vi "4Pi PR.vi"(7 "Calling VI Ref":refnum<vi>) -> ()   [LabVIEW 2021]
uses:
  <vilib>/Utility/miscctls.llb/LVPointTypeDef.ctl
  4Pi Dual DM Control/4Pi Dual DM - Controls/4Pi Dual DM - Standard Action.ctl
  <vilib>/Utility/file.llb/Read Delimited Spreadsheet (DBL).vi
panel:
  in  "Update DM":bool
  out "Spherical":sgl=1.0 format="%.3g"
  out "Coma (x)":sgl=1.0 format="%.3g"
  out "Coma (y)":sgl=1.0 format="%.3g"
  out "Astigmatsim":sgl=1.0 format="%.3g"
  out "Astigmatsim (diag)":sgl=1.0 format="%.3g"
  out "phase plot":cluster{u16[], sgl[]}(graph)
  in  "p factor":dbl=1.0
  in  "Quit":bool
  in  "Start PR":bool
  in  "objective":u16(ring) items=["Bottom", "Top"]
  in  "channel":u16(ring) items=["600", "676"]
  in  "gain":dbl=2.0
  in  "CCD offset":dbl=100.0
  in  "z range (µm)":dbl[](array[numeric])=[-1.0, 1.0, 0.2]
  in  "pixel size  (µm)":dbl=0.129
  in  "refractive index":dbl=1.406
  in  "NA":dbl=1.35
  # "z (µm)[start, end, step]"
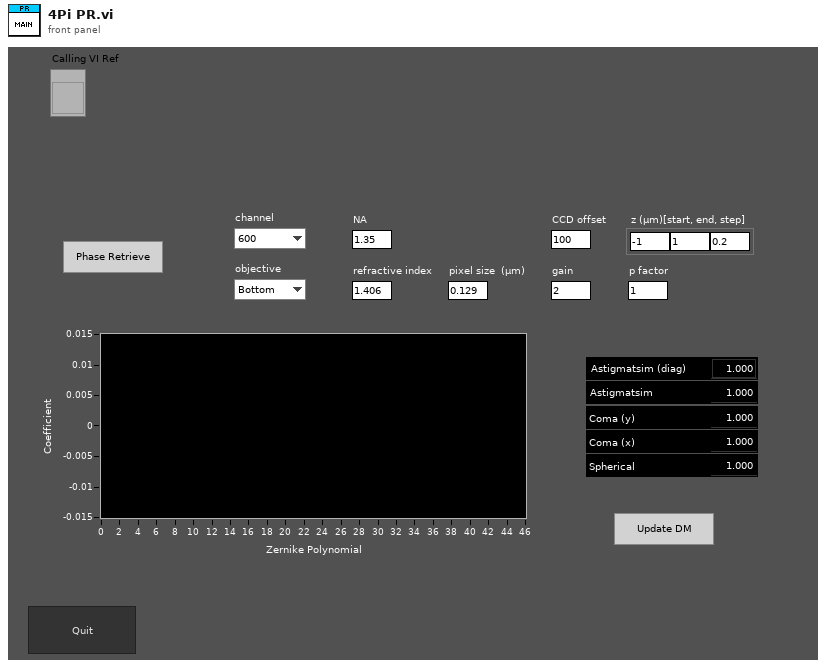
[diagram p1: front panel]
types:
  T1 = enum16{"Always On", "Always Off", "Off While Running"}
  T2 = typedef "LVPointTypeDef.ctl" = cluster{"Horizontal":i16, "Vertical":i16}
  T3 = typedef "4Pi Dual DM - Standard Action.ctl" = enum16{"Read", "Write"}
  T4 = typedef "4Pi Dual DM - Mirror Modes DUAL.ctl" = cluster{"Mode":string, "Amplitude":dbl}[][]
  T5 = typedef "LVRectTypeDef.ctl" = cluster{"Left":i16, "Top":i16, "Right":i16, "Bottom":i16}
  T6 = typedef "LVBoundsTypeDef.ctl" = cluster{"Width":u32, "Height":u32}
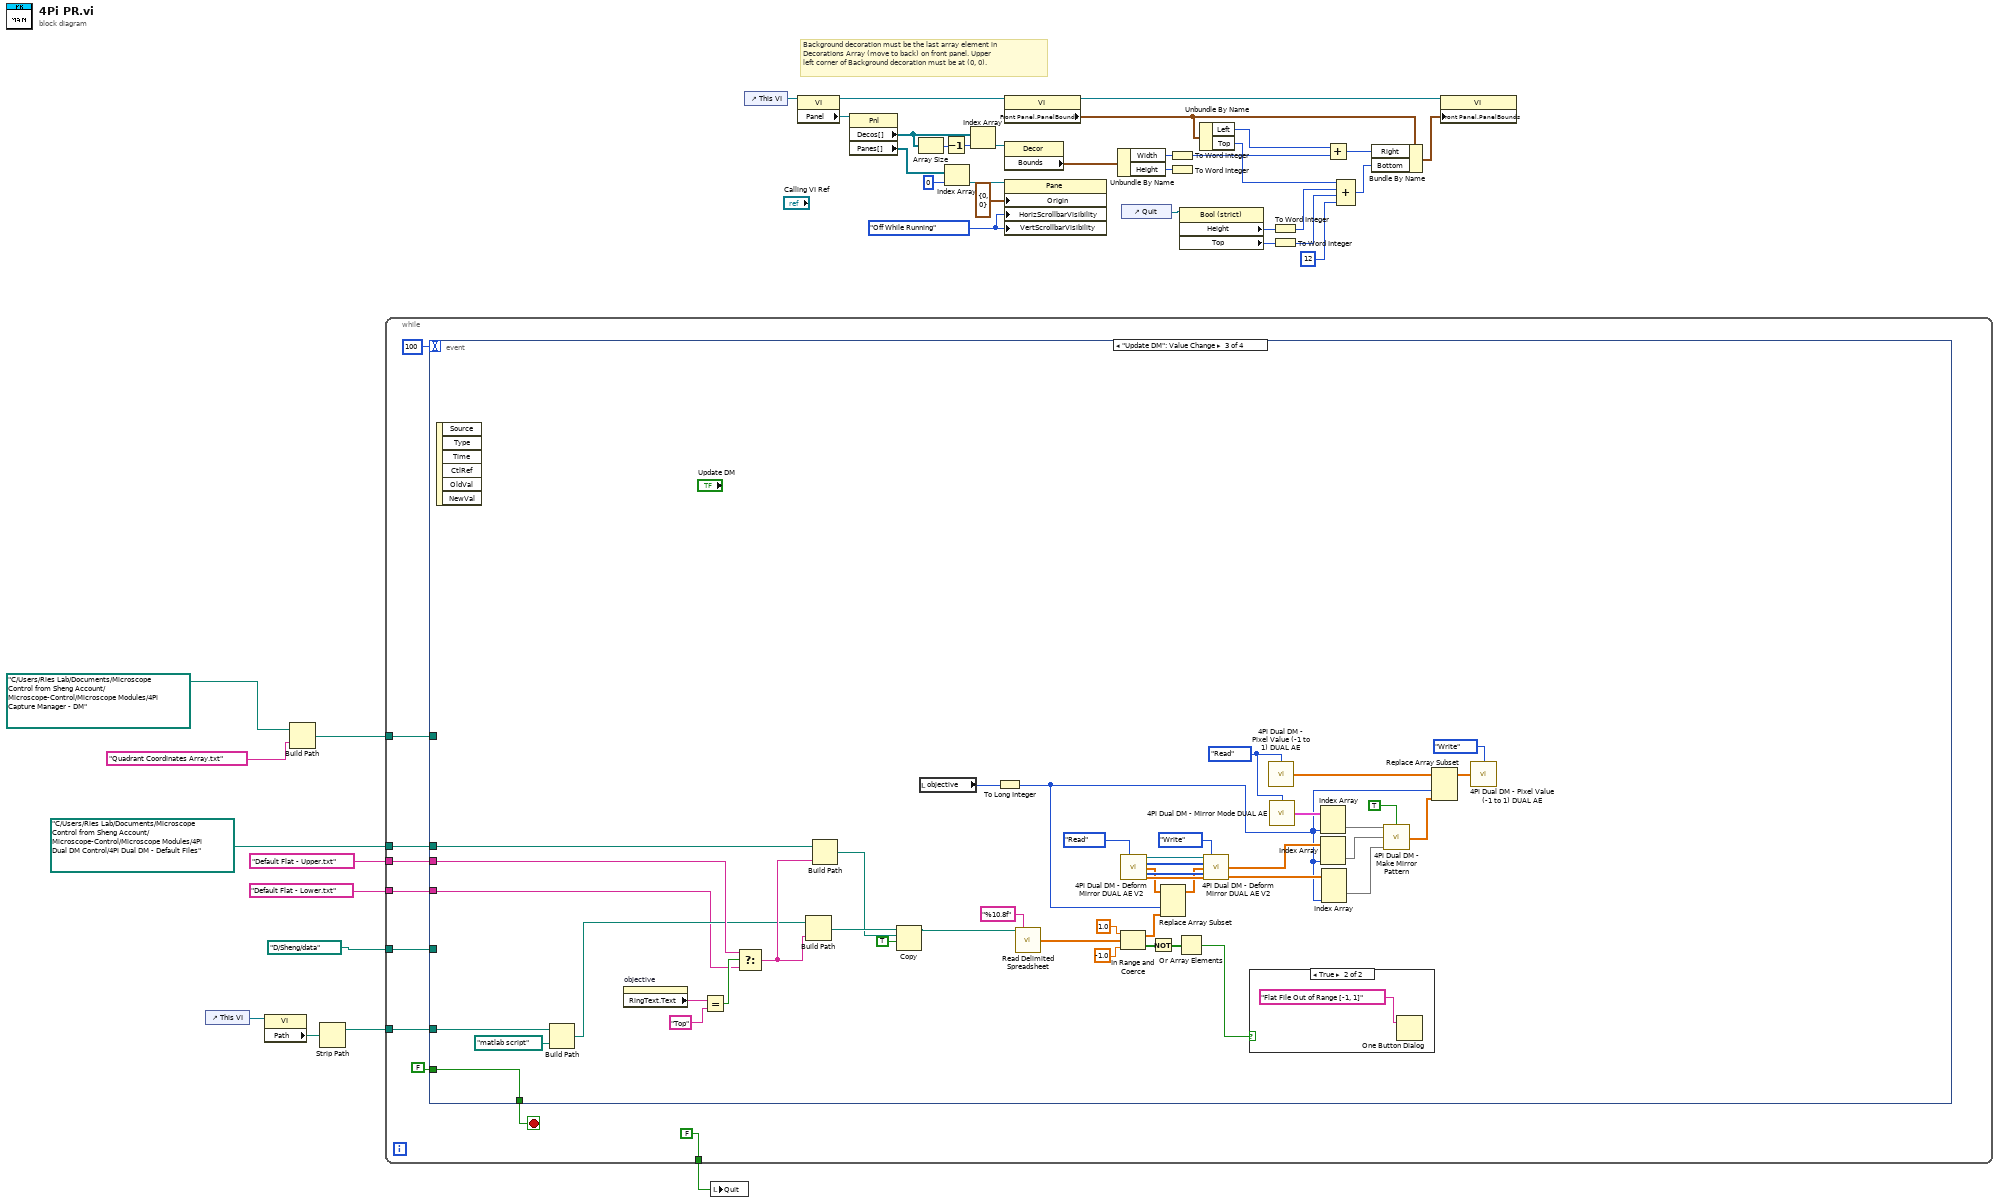
[diagram p0: block diagram]
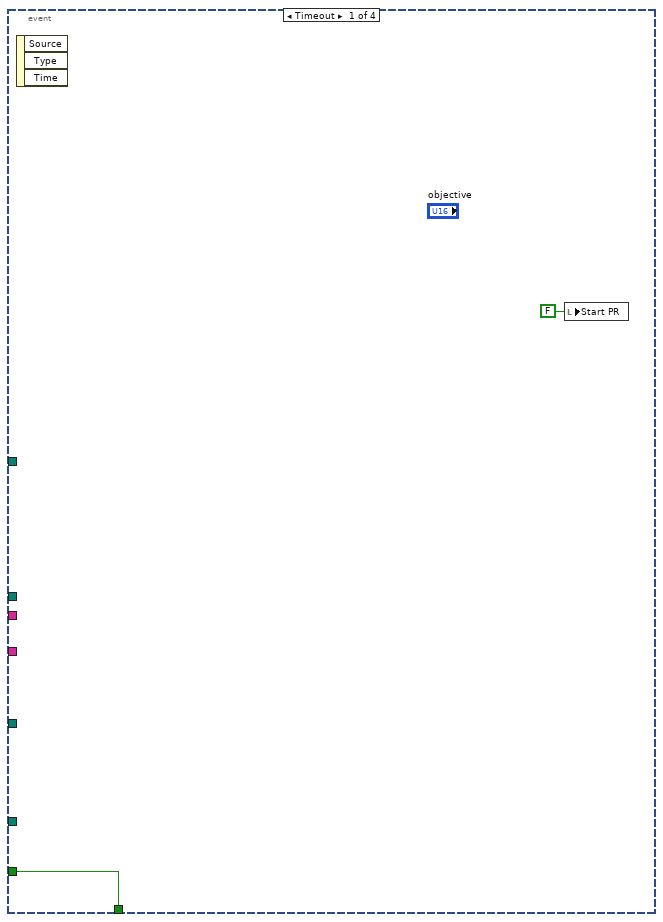
[diagram p2: hidden frame]
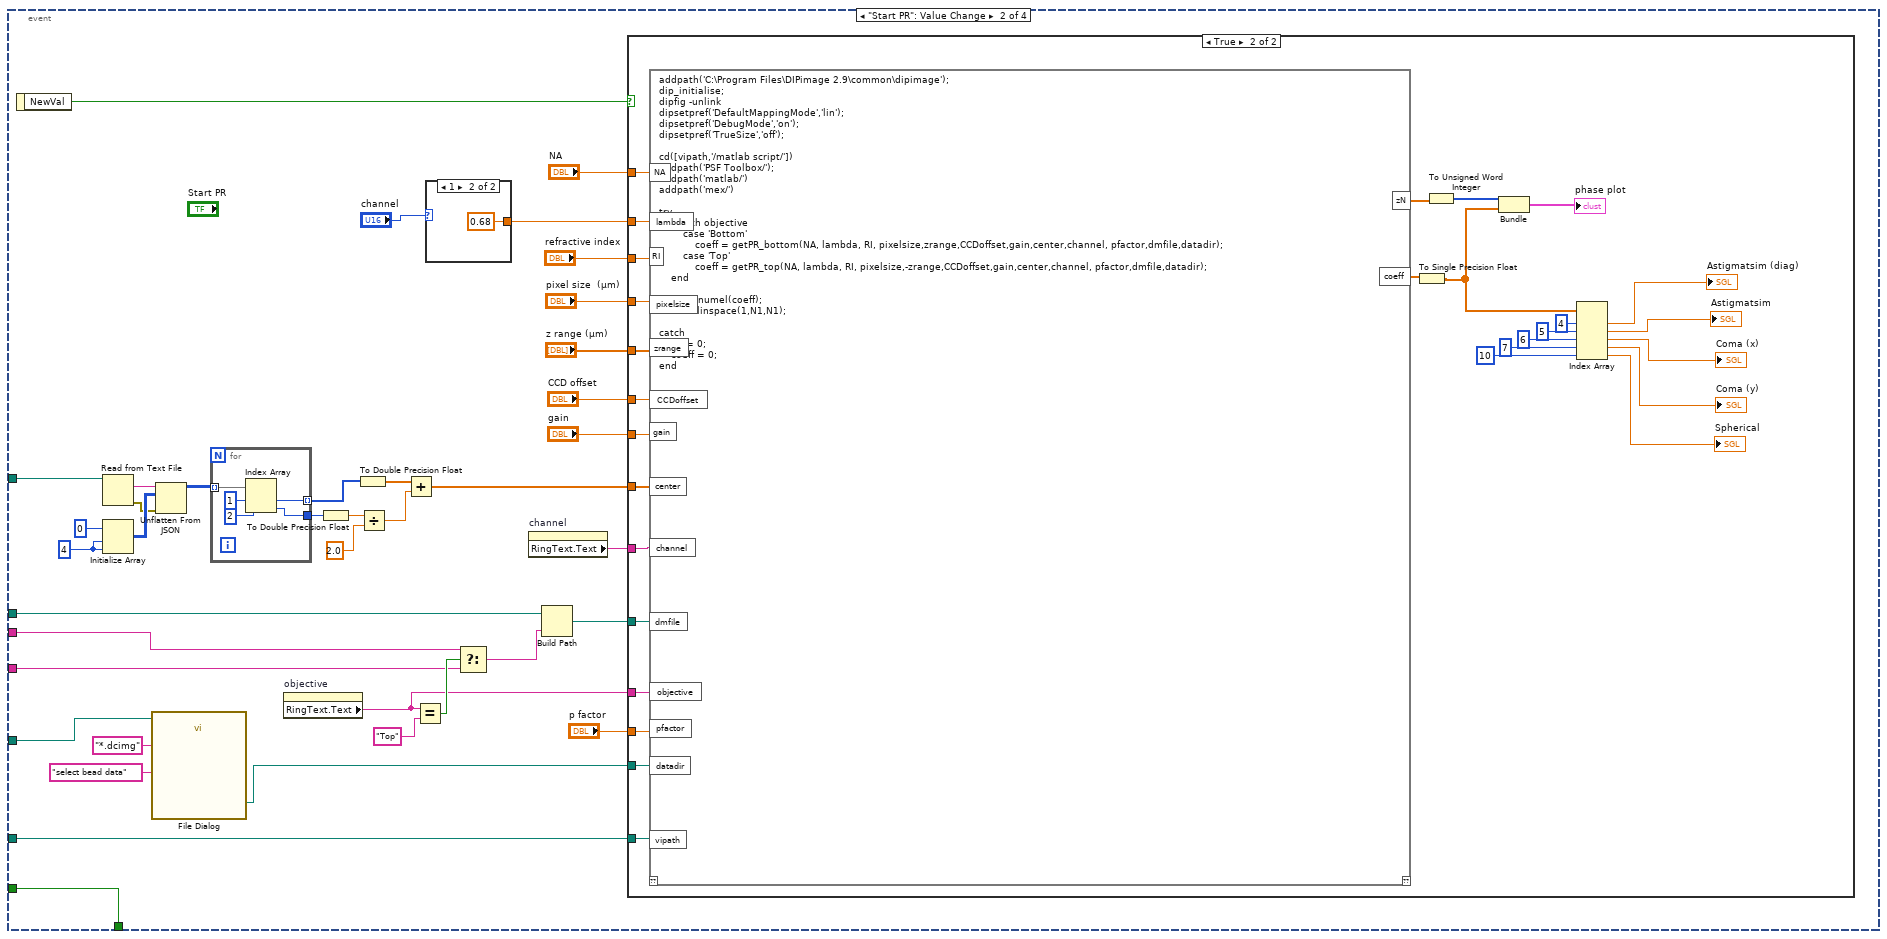
[diagram p3: hidden frame]
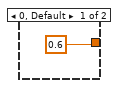
[diagram p4: hidden frame]
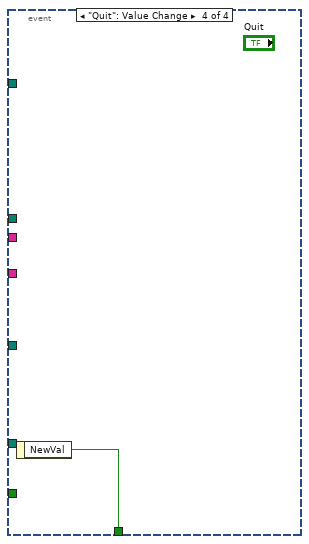
[diagram p7: hidden frame]
diagram:
  w16 = T1."Off While Running" ("Vertical Scrollbar Visibility")
  # "Background decoration must be the last array element in\nDecorations Array (move to back) on front panel. Upper\nleft corner of Background decoration must be at (0, 0)."
  n1 = control-ref of="This VI"() -> (w4:refnum<vi>)
  n2 = property class="VI"(reference=w4) -> ("Path"=w3:path)  [unwired: 1 in, 2 out]
  n3 = Build Path(base path=path "C:/Users/Ries Lab/Documents/Microscope Control from Sheng Account/Microscope-Control/Microscope Modules/4Pi Capture Manager - DM" ("path"), name or relative path="Quadrant Coordinates Array.txt") -> (appended path=w39:path)
  n4 = Strip Path(path=w3) -> (stripped path=w2:path)  [unwired: 1 out]
  n5 = while {
    tunnel: w39 -> [w50]
    tunnel: path "C:/Users/Ries Lab/Documents/Microscope Control from Sheng Account/Microscope-Control/Microscope Modules/4Pi Dual DM Control/4Pi Dual DM - Default Files" ("path") -> [w49]
    tunnel: "Default Flat - Upper.txt" -> [w48]
    tunnel: "Default Flat - Lower.txt" -> [w47]
    tunnel: [FALSE ("Quit")] -> w34
    tunnel: w2 -> [w42]
    tunnel: path "D:/Sheng/data" ("start path") -> [w41]
    stop <- w45 stop-if-true
    n6 = event shown="[2] \"Update DM\": Value Change" {
      selector: _ -> [_ _ _ _]
      dyn-events: _ -> [_ _ _ _]
      timeout: 100 ("Numeric") -> [_ _ _ _]
      tunnel: w50 -> [_ w88 _ _]
      tunnel: w49 -> [_ w77 w151 _]
      tunnel: w48 -> [_ w67 w153 _]
      tunnel: w47 -> [_ w66 w129 _]
      tunnel: [w51 w61 w133 w174] -> w45
      tunnel: FALSE -> [w51 w61 w133 _]
      tunnel: w42 -> [_ w60 w131 _]
      tunnel: w41 -> [_ w59 _ _]
      event Timeout {
        n7 = event-data() -> ()  [unwired: 1 in, 3 out]
        n8 = local write "Start PR"(FALSE ("Start PR")) -> ()
      }
      event "Start PR": Value Change {
        w85 = 4 ("dimension size")
        n9 = event-data() -> ("NewVal"=w62:bool)  [unwired: 1 in]
        n10 = Read from Text File(file (use dialog)=w88) -> (text=w87:string, error out=w86:errorcluster)  [unwired: 3 in, 2 out]
        n11 = Initialize Array(0 ("element"), w85, w85) -> (w89:i32[][])
        n12 = call "File Dialog"("start path"=w59, "prompt"="select bead data", "pattern (all files)"="*.dcimg") -> ("selected path"=w56:path)  [unwired: 9 in, 3 out]
        n13 = Unflatten From JSON(JSON string=w87, type and defaults=w89, error in (no error)=w86) -> (value=w84:i32[][])  [unwired: 4 in, 1 out]
        n14 = for {
          tunnel: w84 -> [w127] mode=indexing
          tunnel: [w125] -> w80 mode=indexing
          tunnel: [w123] -> w83
          n15 = Index Array(array=w127, index #1=1 ("index (row)"), index #2=2 ("index")) -> (element #1=w125:i32, element #2=w123:i32)
        }
        n16 = property on="objective" class="Ring (strict)"() -> ("RingText.Text"=w65:string)  [unwired: 2 in, 2 out]
        n17 = To Double Precision Float(number=w83) -> (double precision float=w82:dbl)
        n18 = To Double Precision Float(number=w80) -> (double precision float=w79:dbl[])
        n19 = Divide(x=w82, y=2.0) -> (x/y=w78:dbl)
        n20 = Add(x=w79, y=w78) -> (x+y=w71:dbl[])
        n21 = Equal?(x=w65, y="Top" ("x")) -> (x = y?=w68:bool)
        n22 = case shown="1" "channel" {
          tunnel: [0.6 ("NA") 0.68 ("NA")] -> w53
          frame 0, Default {
          }
          frame 1 {
          }
        }
        n23 = Select(t=w67, s=w68, f=w66) -> (s? t:f=w63:string)
        n24 = property on="channel" class="Ring (strict)"() -> ("RingText.Text"=w69:string)  [unwired: 2 in, 2 out]
        n25 = Build Path(base path=w77, name or relative path=w63) -> (appended path=w70:path)
        n26 = case shown="True" w62 {
          tunnel: "NA" -> [_ w122]
          tunnel: "refractive index" -> [_ w121]
          tunnel: "pixel size  (µm)" -> [_ w120]
          tunnel: "z range (µm)" -> [_ w119]
          tunnel: "CCD offset" -> [_ w118]
          tunnel: "gain" -> [_ w117]
          tunnel: w71 -> [_ w116]
          tunnel: w70 -> [_ w115]
          tunnel: w56 -> [_ w114]
          tunnel: w69 -> [_ w113]
          tunnel: w65 -> [_ w112]
          tunnel: w60 -> [_ w111]
          tunnel: "p factor" -> [_ w110]
          tunnel: w53 -> [_ w109]
          frame False {
          }
          frame True {
            n27 = script code="addpath('C:\\Program Files\\DIPimage 2.9\\common\\dipimage');\ndip_initialise;\ndipfig -unlink\ndipsetpref('DefaultMappingMode','lin');\ndipsetpref('DebugMode','on');\ndipsetpref('TrueSize','off');\n\ncd([vipath,'/matlab script/'])\naddpath('PSF Toolbox/');\naddpath('matlab/')\naddpath('mex/')\n\ntry\n    switch objective\n        case 'Bottom'\n            coeff = getPR_bottom(NA, lambda, RI, pixelsize,zrange,CCDoffset,gain,center,channel, pfactor,dmfile,datadir);\n        case 'Top'\n            coeff = getPR_top(NA, lambda, RI, pixelsize,-zrange,CCDoffset,gain,center,channel, pfactor,dmfile,datadir);\n    end\n    \n    N1 = numel(coeff);\n    zN = linspace(1,N1,N1);\n    \ncatch\n    zN = 0;\n    coeff = 0;\nend"("NA"=w122, "lambda"=w109, "RI"=w121, "pixelsize"=w120, "zrange"=w119, "CCDoffset"=w118, "gain"=w117, "center"=w116, "channel"=w113, "dmfile"=w115, "datadir"=w114, "objective"=w112, "vipath"=w111, "pfactor"=w110) -> ("coeff"=w95:dbl[], "zN"=w97:dbl[])  [unwired: 1 in, 1 out]
            n28 = To Single Precision Float(number=w95) -> (single precision float=w94:sgl[])
            n29 = To Unsigned Word Integer(number=w97) -> (unsigned 16bit integer=w96:u16[])
            n30 = Bundle(w96, w94) -> (→"phase plot":cluster{u16[], sgl[]})  [unwired: 1 in]
            n31 = Index Array(array=w94, index #1=4 ("index"), index #2=5 ("index"), index #3=6 ("index"), index #4=7 ("index"), index #5=10 ("index")) -> (element #1=→"Astigmatsim (diag)":sgl, element #2=→"Astigmatsim":sgl, element #3=→"Coma (x)":sgl, element #4=→"Coma (y)":sgl, element #5=→"Spherical":sgl)
          }
        }
      }
      event "Update DM": Value Change {
        w144 = 4Pi_Dual_DM_-_Standard_Action."Read" ("Action")
        n32 = event-data() -> ()  [unwired: 1 in, 6 out]
        n33 = Build Path(base path=w131, name or relative path=path "matlab script") -> (appended path=w130:path)
        n34 = property on="objective" class="Ring (strict)"() -> ("RingText.Text"=w154:string)  [unwired: 2 in, 2 out]
        n35 = Equal?(x=w154, y="Top" ("x")) -> (x = y?=w156:bool)
        n36 = Select(t=w153, s=w156, f=w129) -> (s? t:f=w150:string)
        n37 = Build Path(base path=w130, name or relative path=w150) -> (appended path=w152:path)
        n38 = Build Path(base path=w151, name or relative path=w150) -> (appended path=w149:path)
        n39 = Copy(9:TRUE ("overwrite (F)"), 10:w149, 11:w152) -> (3:w148:path)  [unwired: 2 in, 2 out]
        n40 = local read "objective"() -> (w138:u16)
        n41 = To Long Integer(number=w138) -> (32bit integer=w134:i32)
        n42 = call-poly <vilib>:"Read Delimited Spreadsheet.vi"("file path (dialog if empty)"=w148, "format (%.3f)"="%10.8f") -> ("first row"=w162:dbl[])  [unwired: 8 in, 5 out]
        n43 = In Range and Coerce(upper limit=1.0, x=w162, lower limit=-1.0) -> (coerced(x)=w172:dbl[], In Range?=w163:bool[])
        n44 = call "4Pi Dual DM - Deform Mirror DUAL AE V2.vi"("Action"=4Pi_Dual_DM_-_Standard_Action."Read") -> ("Refnum Out"=w171:refnum<k7>, "IDs Out"=w170:i32[], "Flat Files Out"=w167:dbl[][], "Multi Map Data Out"=w169:i32[], "Mode Matrix Out"=w168:dbl[][][])  [unwired: 10 in]
        n45 = Not(x=w163) -> (.not. x?=w164:bool[])
        n46 = Replace Array Subset(array=w167, new element=w172, index (col)=w134) -> (w166:dbl[][])  [unwired: 1 in]
        n47 = Or Array Elements(Boolean array=w164) -> (logical OR=w165:bool)
        n48 = call "4Pi Dual DM - Deform Mirror DUAL AE V2.vi"("Refnum In"=w171, "Action"=4Pi_Dual_DM_-_Standard_Action."Write", "IDs In"=w170, "Flat Files In"=w166, "Multi Map Data In"=w169, "Mode Matrix"=w168) -> ("Flat Files Out"=w135:dbl[][], "Mode Matrix Out"=w136:dbl[][][])  [unwired: 5 in, 3 out]
        n49 = case shown="True" w165 {
          frame False {
          }
          frame True {
            n50 = One Button Dialog(message="Flat File Out of Range [-1, 1]") -> ()  [unwired: 1 in, 1 out]
          }
        }
        n51 = call "4Pi Dual DM - Pixel Value (-1 to 1) DUAL AE.vi"("Action"=w144) -> ("Pixel Value (-1 to 1) Out"=w145:dbl[][])  [unwired: 14 in]
        n52 = call "4Pi Dual DM - Mirror Mode DUAL AE.vi"("Action"=w144) -> ("Mirror Modes Out"=w141:T4)  [unwired: 14 in]
        n53 = Index Array(array=w141, index (col)=w134) -> (element=w142:cluster{"Mode":string, "Amplitude":dbl}[])  [unwired: 1 in]
        n54 = Index Array(array=w135, index (col)=w134) -> (element=w140:dbl[])  [unwired: 1 in]
        n55 = Index Array(array=w136, index (dim 2)=w134) -> (element=w139:dbl[][])  [unwired: 2 in]
        n56 = call "4Pi Dual DM - Make Mirror Pattern.vi"("Mirror Modes In"=w142, "Flat On?"=TRUE, "Flat File In"=w140, "Mirror Modes Array"=w139) -> ("Pixel Value U (-1 to 1)"=w146:dbl[])  [unwired: 11 in]
        n57 = Replace Array Subset(array=w145, new element=w146, index (col)=w134) -> (w147:dbl[][])  [unwired: 1 in]
        n58 = call "4Pi Dual DM - Pixel Value (-1 to 1) DUAL AE.vi"("Action"=4Pi_Dual_DM_-_Standard_Action."Write", "Pixel Value (-1 to 1)"=w147) -> ()  [unwired: 13 in, 1 out]
      }
      event "Quit": Value Change {
        n59 = event-data() -> ("NewVal"=w174:bool)  [unwired: 1 in]
      }
    }
  }
  n60 = local write "Quit"(w34) -> ()
  n61 = control-ref of="This VI"() -> (w9:refnum<vi>)
  n62 = property class="VI"(reference=w9) -> (reference out=w17:refnum<vi>, "Panel"=w10:refnum<vi>)  [unwired: 1 in, 1 out]
  n63 = property class="Pnl"(reference=w10) -> ("Decos[]"=w8:refnum<vi>[], "Panes[]"=w13:refnum<vi>[])  [unwired: 1 in, 2 out]
  n64 = Array Size(array=w8) -> (size(s)=w6:i32)
  n65 = Decrement(x=w6) -> (x-1=w7:i32)
  n66 = Index Array(array=w13, index=0) -> (element=w12:refnum<vi>)
  n67 = Index Array(array=w8, index=w7) -> (element=w15:refnum<vi>)
  n68 = property class="VI"(reference=w17) -> (reference out=w19:refnum<vi>, "Front Panel.PanelBounds"=w20:T5)  [unwired: 1 in, 1 out]
  n69 = property class="Decor"(reference=w15) -> ("Bounds"=w18:T6)  [unwired: 1 in, 2 out]
  n70 = property class="Pane"(reference=w12, "Origin"=T2 {"Horizontal"=0, "Vertical"=0}, "HorizScrollbarVisibility"=w16, "VertScrollbarVisibility"=w16) -> ()  [unwired: 1 in, 2 out]
  n71 = Unbundle By Name(w18) -> ("Width"=w23:u32, "Height"=w26:u32)
  n72 = control-ref of="Quit"() -> (w5:refnum<vi>)
  n73 = To Word Integer(number=w23) -> (16bit integer=w25:i16)
  n74 = To Word Integer(number=w26) -> ()  [unwired: 1 out]
  n75 = property class="Bool (strict)"(reference=w5) -> ("Height"=w28:u32, "Top"=w29:i32)  [unwired: 1 in, 2 out]
  n76 = Unbundle By Name(w20) -> ("Left"=w22:i16, "Top"=w33:i16)
  n77 = To Word Integer(number=w28) -> (16bit integer=w31:i16)
  n78 = To Word Integer(number=w29) -> (16bit integer=w32:i16)
  n79 = Add(x=w22, y=w25) -> (x+y=w24:i16)
  n80 = Compound Arithmetic op=ADD(w33, w31, w32, i16 12 ("y")) -> (w27:i16)
  n81 = Bundle By Name(cluster=w20, "Right"=w24, "Bottom"=w27) -> (w21:T5)
  n82 = property class="VI"(reference=w19, "Front Panel.PanelBounds"=w21) -> ()  [unwired: 1 in, 2 out]
